vi "oa_Get N Cycle of Even Angle Signal.vi"(7 "reset":bool, 8 "new even angle signal":cluster{"r0":dbl, "dr":dbl, "Y":dbl[]}={"r0"=0.0, "dr"=1.0, "Y"=[]} {"r0" format="%.2p"; "dr" format="%.2p"; "Y" format="%.2f"}, 9 "averaging revolution (1)":dbl=1.0 min=0.0, 11 "rest even angle signal":cluster{"r0":dbl, "dr":dbl, "Y":dbl[]}={"r0"=0.0, "dr"=1.0, "Y"=[]} {"r0" format="%.2p"; "dr" format="%.2p"; "Y" format="%.2f"}) -> (0 "data for averaging":dbl[](array[numeric]), 1 "number of averages":dbl, 2 "even angle signal":cluster{"r0":dbl, "dr":dbl, "Y":dbl[]}, 3 "rest even angle signal out":cluster{"r0":dbl, "dr":dbl, "Y":dbl[]})   [LabVIEW 2017, in "SoundVib_OAUtility.lvlib"]
uses:
  <vilib>/addons/Sound and Vibration/Order Analysis/Utility/SoundVib_OAUtility.lvlib
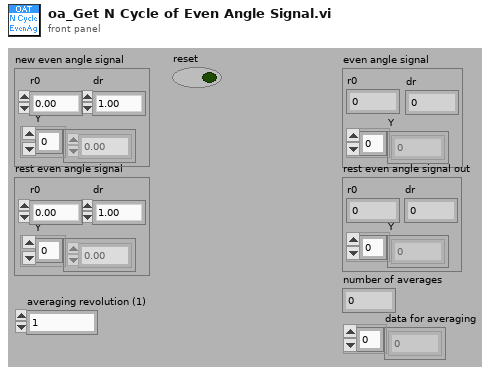
[diagram p1: front panel]
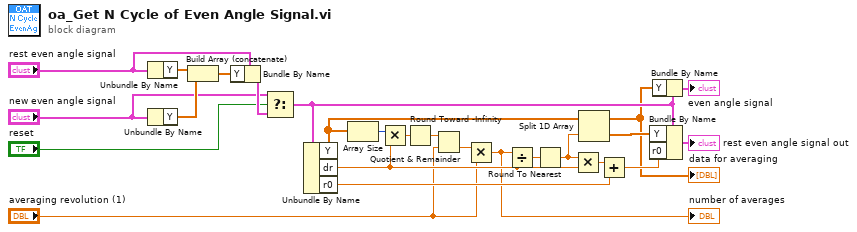
[diagram p0: block diagram]
diagram:
  n1 = Unbundle By Name("rest even angle signal") -> ("Y"=w25:dbl[])
  n2 = Unbundle By Name("new even angle signal") -> ("Y"=w24:dbl[])
  n3 = Build Array (concatenate)(w25, w24) -> (w23:dbl[])
  n4 = Bundle By Name(cluster="rest even angle signal", "Y"=w23) -> (w22:cluster{"r0":dbl, "dr":dbl, "Y":dbl[]})
  n5 = Select(t="new even angle signal", s="reset", f=w22) -> (s? t:f=w7:cluster{"r0":dbl, "dr":dbl, "Y":dbl[]})
  n6 = Unbundle By Name(w7) -> ("Y"=w15:dbl[], "dr"=w12:dbl, "r0"=w17:dbl)
  n7 = Array Size(array=w15) -> (size(s)=w21:i32)
  n8 = Multiply(x=w21, y=w12) -> (x*y=w20:dbl)
  n9 = Round Toward -Infinity(1:w20) -> (0:w4:dbl)
  n10 = Quotient & Remainder(x=w4, y="averaging revolution (1)") -> (floor(x/y)=w3:dbl)  [unwired: 1 out]
  n11 = Multiply(x=w3, y="averaging revolution (1)") -> (x*y=w1:dbl)
  "number of averages" <- w1
  n12 = Divide(x=w1, y=w12) -> (x/y=w19:dbl)
  n13 = Round To Nearest(number=w19) -> (nearest integer value=w14:dbl)
  n14 = Multiply(x=w14, y=w12) -> (x*y=w18:dbl)
  n15 = Split 1D Array(array=w15, index=w14) -> (first subarray=w5:dbl[], second subarray=w13:dbl[])
  "data for averaging" <- w5
  n16 = Add(x=w18, y=w17) -> (x+y=w16:dbl)
  n17 = Bundle By Name(cluster=w7, "Y"=w13, "r0"=w16) -> (→"rest even angle signal out":cluster{"r0":dbl, "dr":dbl, "Y":dbl[]})
  n18 = Bundle By Name(cluster=w7, "Y"=w5) -> (→"even angle signal":cluster{"r0":dbl, "dr":dbl, "Y":dbl[]})
